vi "Mean_and_Variance_Stats.vi"(4 "Block No":i32=1, 5 "Shift in":dbl[](array[numeric]) format="%.2f", 8 "U":dbl[](array[numeric]) format="%.2f") -> (0 "Shift out":dbl[](array[numeric]) format="%.2f", 2 "u^2":dbl, 3 "U":dbl)   [LabVIEW 2014]
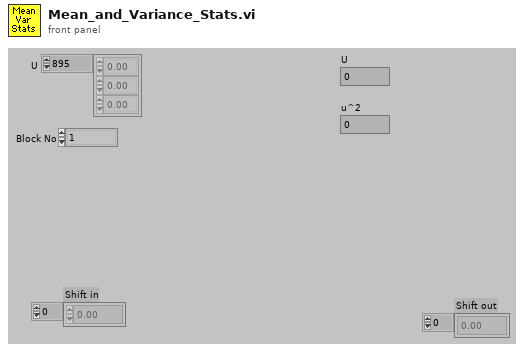
[diagram p1: front panel]
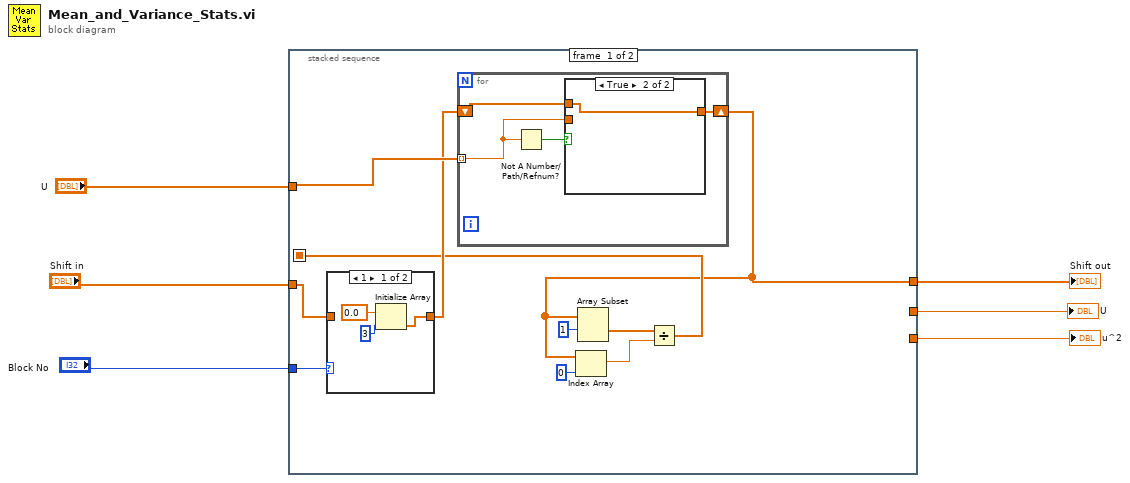
[diagram p0: block diagram]
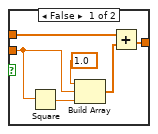
[diagram p3: hidden frame]
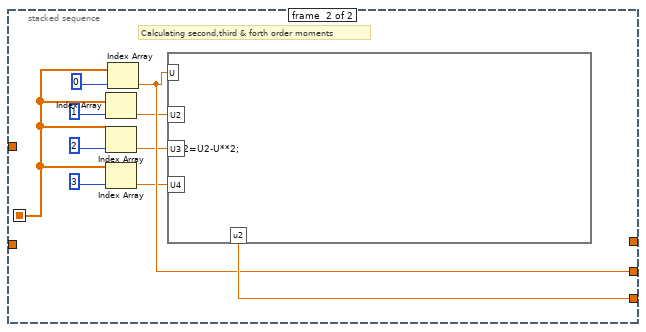
[diagram p4: hidden frame]
diagram:
  n1 = stacked-sequence {
    seq-local: [w8 _] -> [_ w39]
    tunnel: "U" -> [w16 _]
    tunnel: [w7 _] -> w5
    tunnel: "Shift in" -> [w10 _]
    tunnel: "Block No" -> [w11 _]
    tunnel: [_ w35] -> w2
    tunnel: [_ w36] -> w1
    frame #0 {
      n2 = case shown="1" w11 {
        tunnel: [w17 w20] -> w9
        tunnel: w10 -> [_ w20]
        frame 1 {
          n3 = Initialize Array(0.0 ("Element Data"), 3 ("Dimension Size")) -> (w17:dbl[])
        }
        frame 2, Default {
        }
      }
      n4 = for {
        shift-right: [w23] -> w7
        shift-left: w9 -> [w24]
        tunnel: w16 -> [w22] mode=indexing
        n5 = Not A Number/Path/Refnum?(number/path/refnum=w22) -> (NaN/Path/Refnum?=w21:bool)
        n6 = case shown="True" w21 {
          tunnel: w24 -> [w30 w31]
          tunnel: [w29 w31] -> w23
          tunnel: w22 -> [w25 _]
          frame False {
            n7 = Square(x=w25) -> (x^2=w26:dbl)
            n8 = Build Array(1.0 ("Input Element"), w25, w26) -> (w28:dbl[])
            n9 = Add(x=w30, y=w28) -> (x+y=w29:dbl[])
          }
          frame True {
          }
        }
      }
      n10 = Index Array(array=w7, index=0 ("Index")) -> (element=w12:dbl)
      n11 = Array Subset(array=w7, index=1 ("Array Index")) -> (w13:dbl[])  [unwired: 1 in]
      n12 = Divide(x=w13, y=w12) -> (x/y=w8:dbl[])
    }
    frame #1 {
      # "Calculating second,third & forth order moments"
      n13 = Index Array(array=w39, index=1) -> (element=w34:dbl)
      n14 = Index Array(array=w39, index=2) -> (element=w33:dbl)
      n15 = Index Array(array=w39, index=3) -> (element=w32:dbl)
      n16 = Index Array(array=w39, index=0) -> (element=w35:dbl)
      n17 = formula code="u2=U2-U**2;"("U"=w35, "U2"=w34, "U3"=w33, "U4"=w32) -> ("u2"=w36:dbl)
    }
  }
  "Shift out" <- w5
  "U" <- w2
  "u^2" <- w1
